vi "19-AxisInfo.vi"(11 "Axis":i32[](array[numeric])) -> (3 "Axis Info":T1)   [LabVIEW 2019, in "19.lvlib"]
uses:
  19.lvlib
  <userlib>/_OpenG.lib/array/array.llb/Sort 1D Array (I32)__ogtk.vi
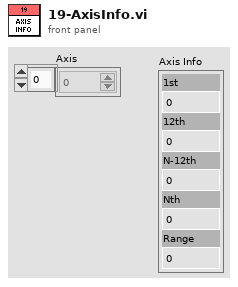
[diagram p1: front panel]
types:
  T1 = cluster{"1st":i32, "12th":i32, "N-12th":i32, "Nth":i32, "Range":i32}
  T2 = cluster{"Numeric":i32, "Numeric":i32, "Numeric":i32, "Numeric":i32, i32}
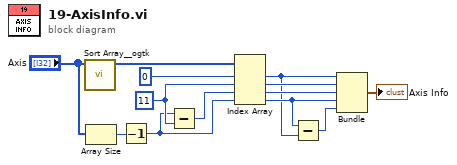
[diagram p0: block diagram]
diagram:
  w7 = 11 ("index")
  n1 = call-poly <userlib>:"Sort Array__ogtk.vi"("Array in"="Axis") -> ("Sorted Array out"=w11:i32[])  [unwired: 9 in, 1 out]
  n2 = Array Size(array="Axis") -> (size(s)=w9:i32)
  n3 = Decrement(x=w9) -> (x-1=w6:i32)
  n4 = Subtract(x=w6, y=w7) -> (x-y=w8:i32)
  n5 = Index Array(array=w11, index #1=0 ("index"), index #2=w7, index #3=w8, index #4=w6) -> (element #1=w1:i32, element #2=w13:i32, element #3=w3:i32, element #4=w5:i32)
  n6 = Subtract(x=w5, y=w1) -> (x-y=w4:i32)
  n7 = Bundle("Numeric"=w1, "Numeric"=w13, "Numeric"=w3, "Numeric"=w5, w4) -> (→"Axis Info":T2)  [unwired: 1 in]
